vi "Read Decorations[].vi"(8 "error in (no error)":errorcluster, 11 "Cluster.lvclass in":refnum<class "Cluster.lvclass">) -> (0 "error out":errorcluster, 2 "Decos[]":refnum<vi>[](array[refnum]), 3 "Cluster.lvclass out":refnum<class "Cluster.lvclass">)   [LabVIEW 2015, in "Cluster.lvclass"]
uses:
  Cluster.lvclass
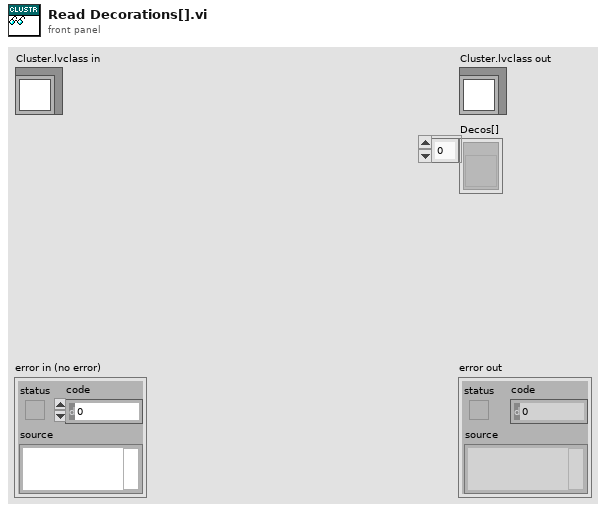
[diagram p1: front panel]
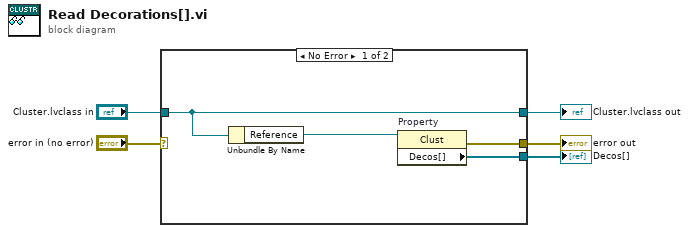
[diagram p0: block diagram]
diagram:
  n1 = case shown="No Error" "error in (no error)" {
    selector: "error in (no error)" -> [_ w11]
    tunnel: [w8 w11] -> w4
    tunnel: [w7 w10] -> w2
    tunnel: "Cluster.lvclass in" -> [w7 w10]
    tunnel: [w9 _] -> w1
    frame No Error {
      n2 = Unbundle By Name(w7) -> ("Reference"=w6:refnum<vi>)
      n3 = property on="Property" class="Clust"(reference=w6) -> (error out=w8:errorcluster, "Decos[]"=w9:refnum<vi>[])  [unwired: 1 in, 1 out]
    }
    frame Error {
    }
  }
  "error out" <- w4
  "Cluster.lvclass out" <- w2
  "Decos[]" <- w1
